vi "Get EM Gain Range.vi"(8 "error in (no error)":errorcluster, 10 "high":i32, 11 "low":i32) -> (0 "error out":errorcluster, 1 "function return":u32, 2 "high out":i32, 3 "low out":i32)   [LabVIEW 2014, in "atmcd32d.lvlib"]
doc: "unsigned int WINAPI GetEMGainRange(int * low, int * high);"
uses:
  atmcd32d.lvlib
  atmcd32d.dll
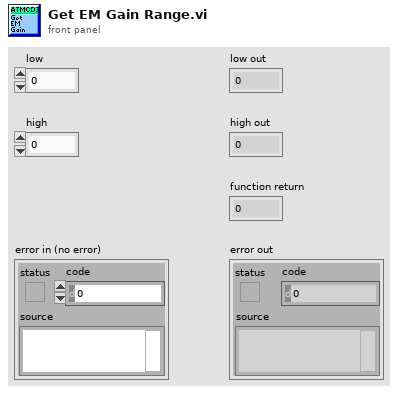
[diagram p1: front panel]
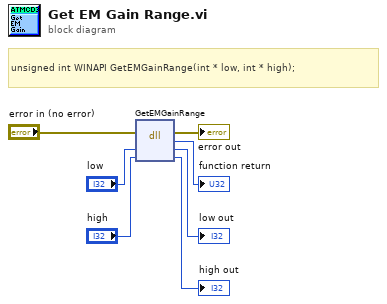
[diagram p0: block diagram]
diagram:
  # "unsigned int WINAPI GetEMGainRange(int * low, int * high);"
  n1 = dll-call lib="C:/Users/Bakir/Documents/Lambda2-Testing/lib/Andorlib/atmcd32d.*" fn="GetEMGainRange"(error in="error in (no error)", "low"="low", "high"="high") -> (error out=→"error out":errorcluster, →"function return":u32, "low"=→"low out":i32, "high"=→"high out":i32)  [unwired: 2 in, 1 out]
